vi "Read Time.vi"(8 "error in (no error)":errorcluster, 11 "ControlDragOverMsg In":refnum<class "ControlDragOverMsg.lvclass">) -> (0 "error out":errorcluster, 2 "Time":u32, 3 "ControlDragOverMsg Out":refnum<class "ControlDragOverMsg.lvclass">)   [LabVIEW 2017, in "ActorEvents.lvlib" / "ControlDragOverMsg.lvclass"]
uses:
  ControlDragOverMsg.lvclass
  ControlDragOverMsg.lvclass/ControlDragOverMsg.ctl
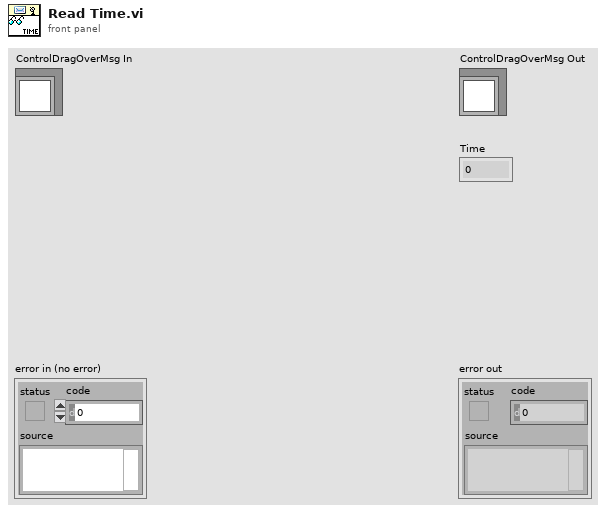
[diagram p1: front panel]
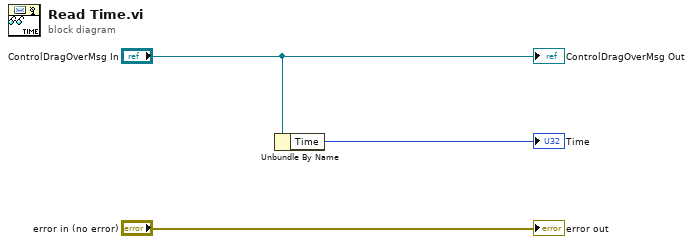
[diagram p0: block diagram]
diagram:
  n1 = Unbundle By Name("ControlDragOverMsg In") -> ("Time"=→"Time":u32)
  "error out" <- "error in (no error)"
  "ControlDragOverMsg Out" <- "ControlDragOverMsg In"
